vi "Autonomous Independent.vi"() -> ()   [LabVIEW 2018]
doc: "This VI is called when autonomous begins, and will automatically be terminated when autonomous ends. You can carry out timed or sensor driven robot movement independently without needing to return to the caller."
uses:
  <vilib>/Rock Robotics/WPI/DriverStation/WPI_DriverStationDerivedRobotMode.ctl
panel:
  out "ENCODER VALUE cLIMBER":dbl=20.0 format="%#_13g"
  out "ENCODER VALUE Retractor":dbl=20.0 format="%#_13g"
  out "ENCODER VALUE LIFT 2":dbl=20.0 format="%#_13g"
  out "ENCODER VALUE LIFT":dbl=20.0 format="%#_13g"
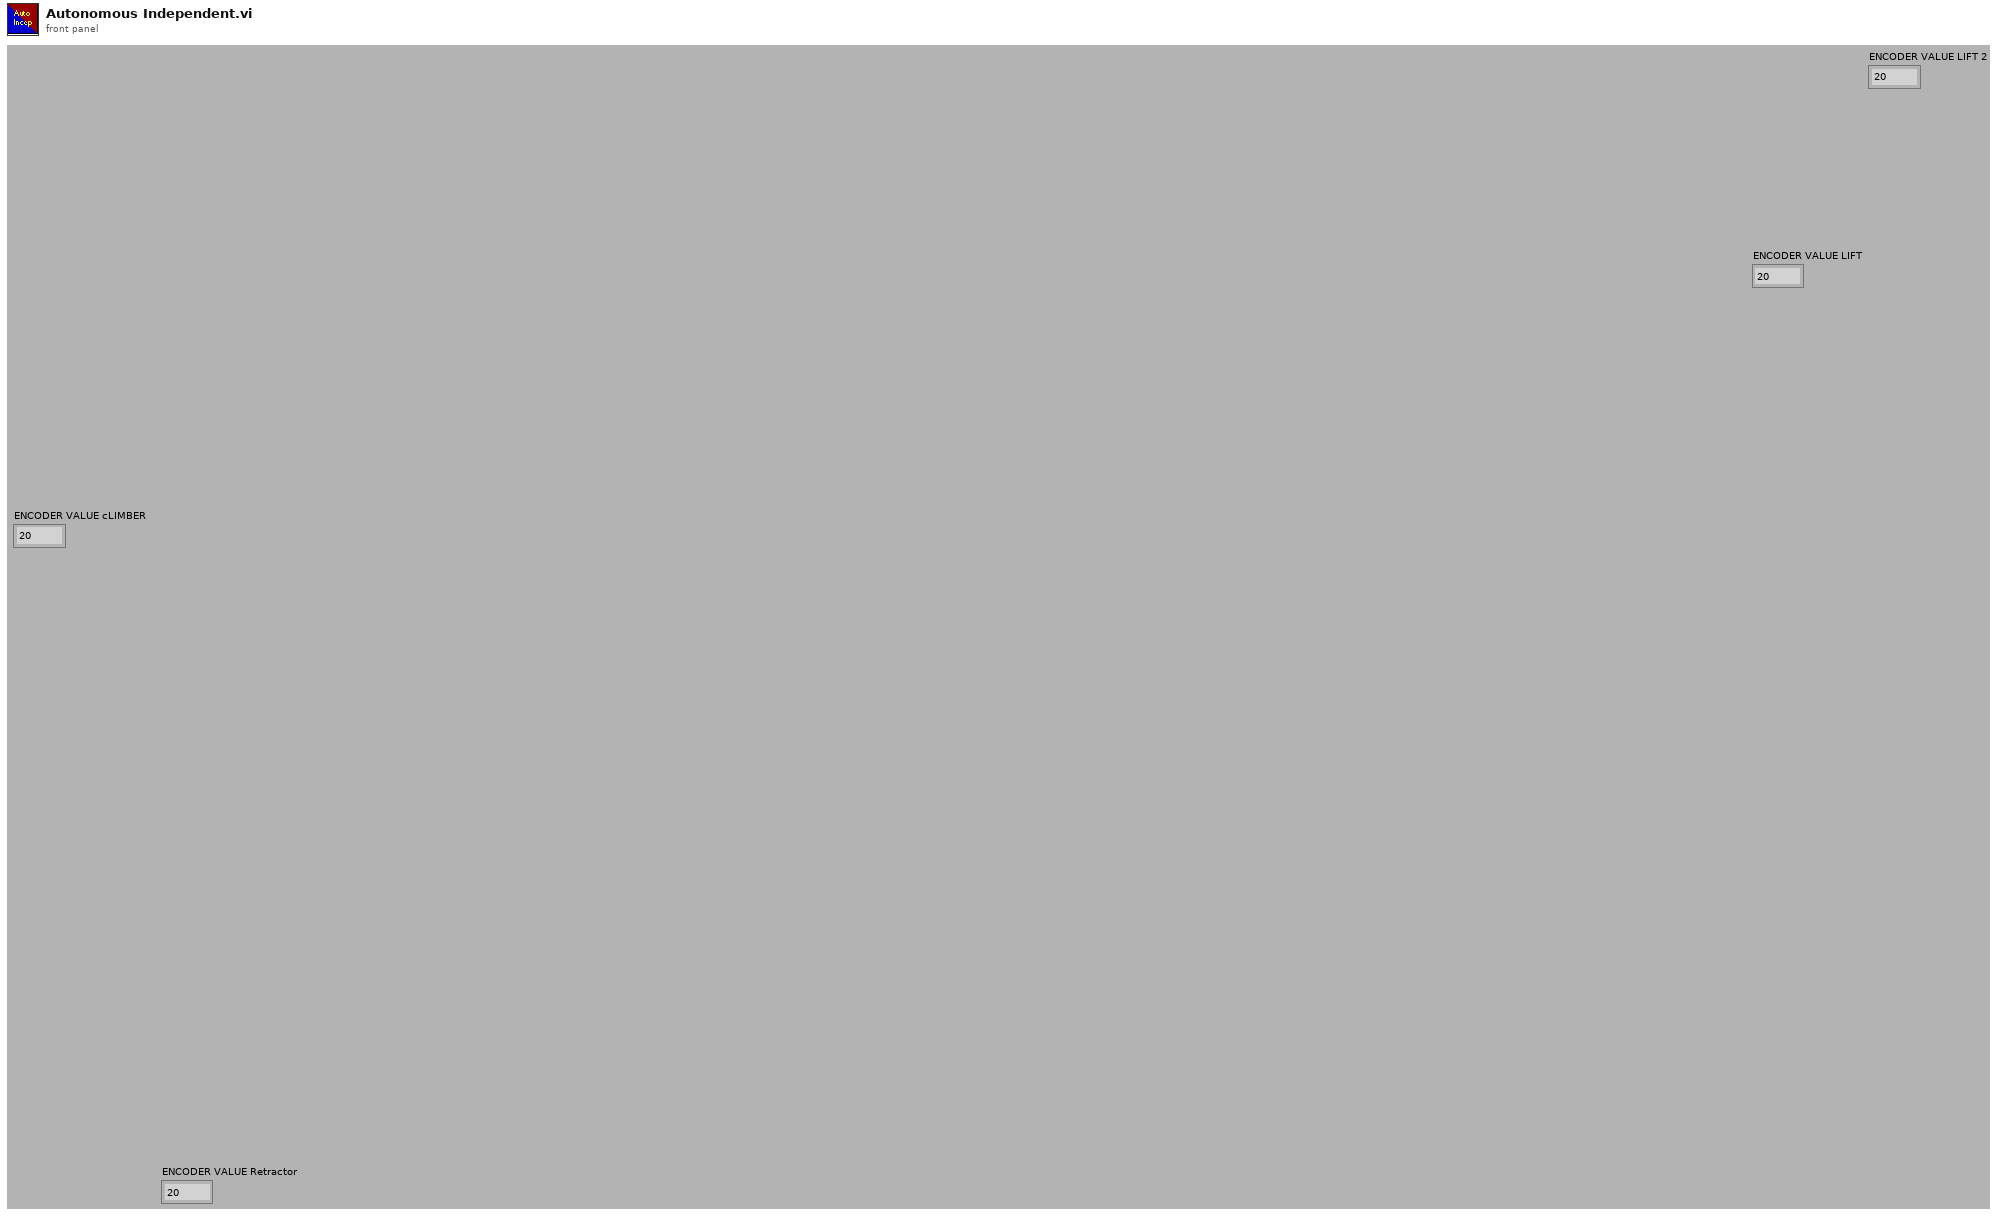
[diagram p1: front panel]
types:
  T1 = typedef "WPI_DriverStationDerivedRobotMode.ctl" = enum16{"Init", "Execute", "Stop"}
  T2 = typedef "WPI_JoystickDevRef.ctl" = cluster{"Device":T3}
  T3 = typedef "WPI_JoystickDeviceEnum.ctl" = enum16{"USB 0", "USB 1", "USB 2", "USB 3", "USB 4", "USB 5"}
  T4 = cluster{"Buttons[0]":bool, "Buttons[1]":bool, "Buttons[2]":bool, "Buttons[3]":bool, "Buttons[4]":bool, "Buttons[5]":bool, "Buttons[6]":bool, "Buttons[7]":bool, "Buttons[8]":bool, "Buttons[9]":bool}
  T5 = cluster{"Buttons[0]":bool, "Buttons[1]":bool, "Buttons[2]":bool, "Buttons[3]":bool, "Buttons[4]":bool, "Buttons[5]":bool, "Buttons[6]":bool, "Buttons[7]":bool, "Buttons[8]":bool, "Buttons[9]":bool, "Buttons[10]":bool, "Buttons[11]":bool}
  T6 = typedef "WPI_EncoderDevRef.ctl" = cluster{"DevStatus":errorcluster, "EncoderIndex":T7, "CounterIndex":T8, "DistancePerCount":dbl, "Decoding Type":T9}
  T7 = typedef "FPGA_EncoderIdx.ctl" = enum8{"Enc 0", "Enc 1", "Enc 2", "Enc 3", "Enc 4", "Enc 5", "Enc 6", "Enc 7", "Invalid"}
  T8 = typedef "FPGA_CounterCtrSystemIndex.ctl" = enum8{"Ctr 0", "Ctr 1", "Ctr 2", "Ctr 3", "Ctr 4", "Ctr 5", "Ctr 6", "Ctr 7", "Invalid"}
  T9 = typedef "WPI_EncoderType.ctl" = enum16{"1x", "2x", "4x"}
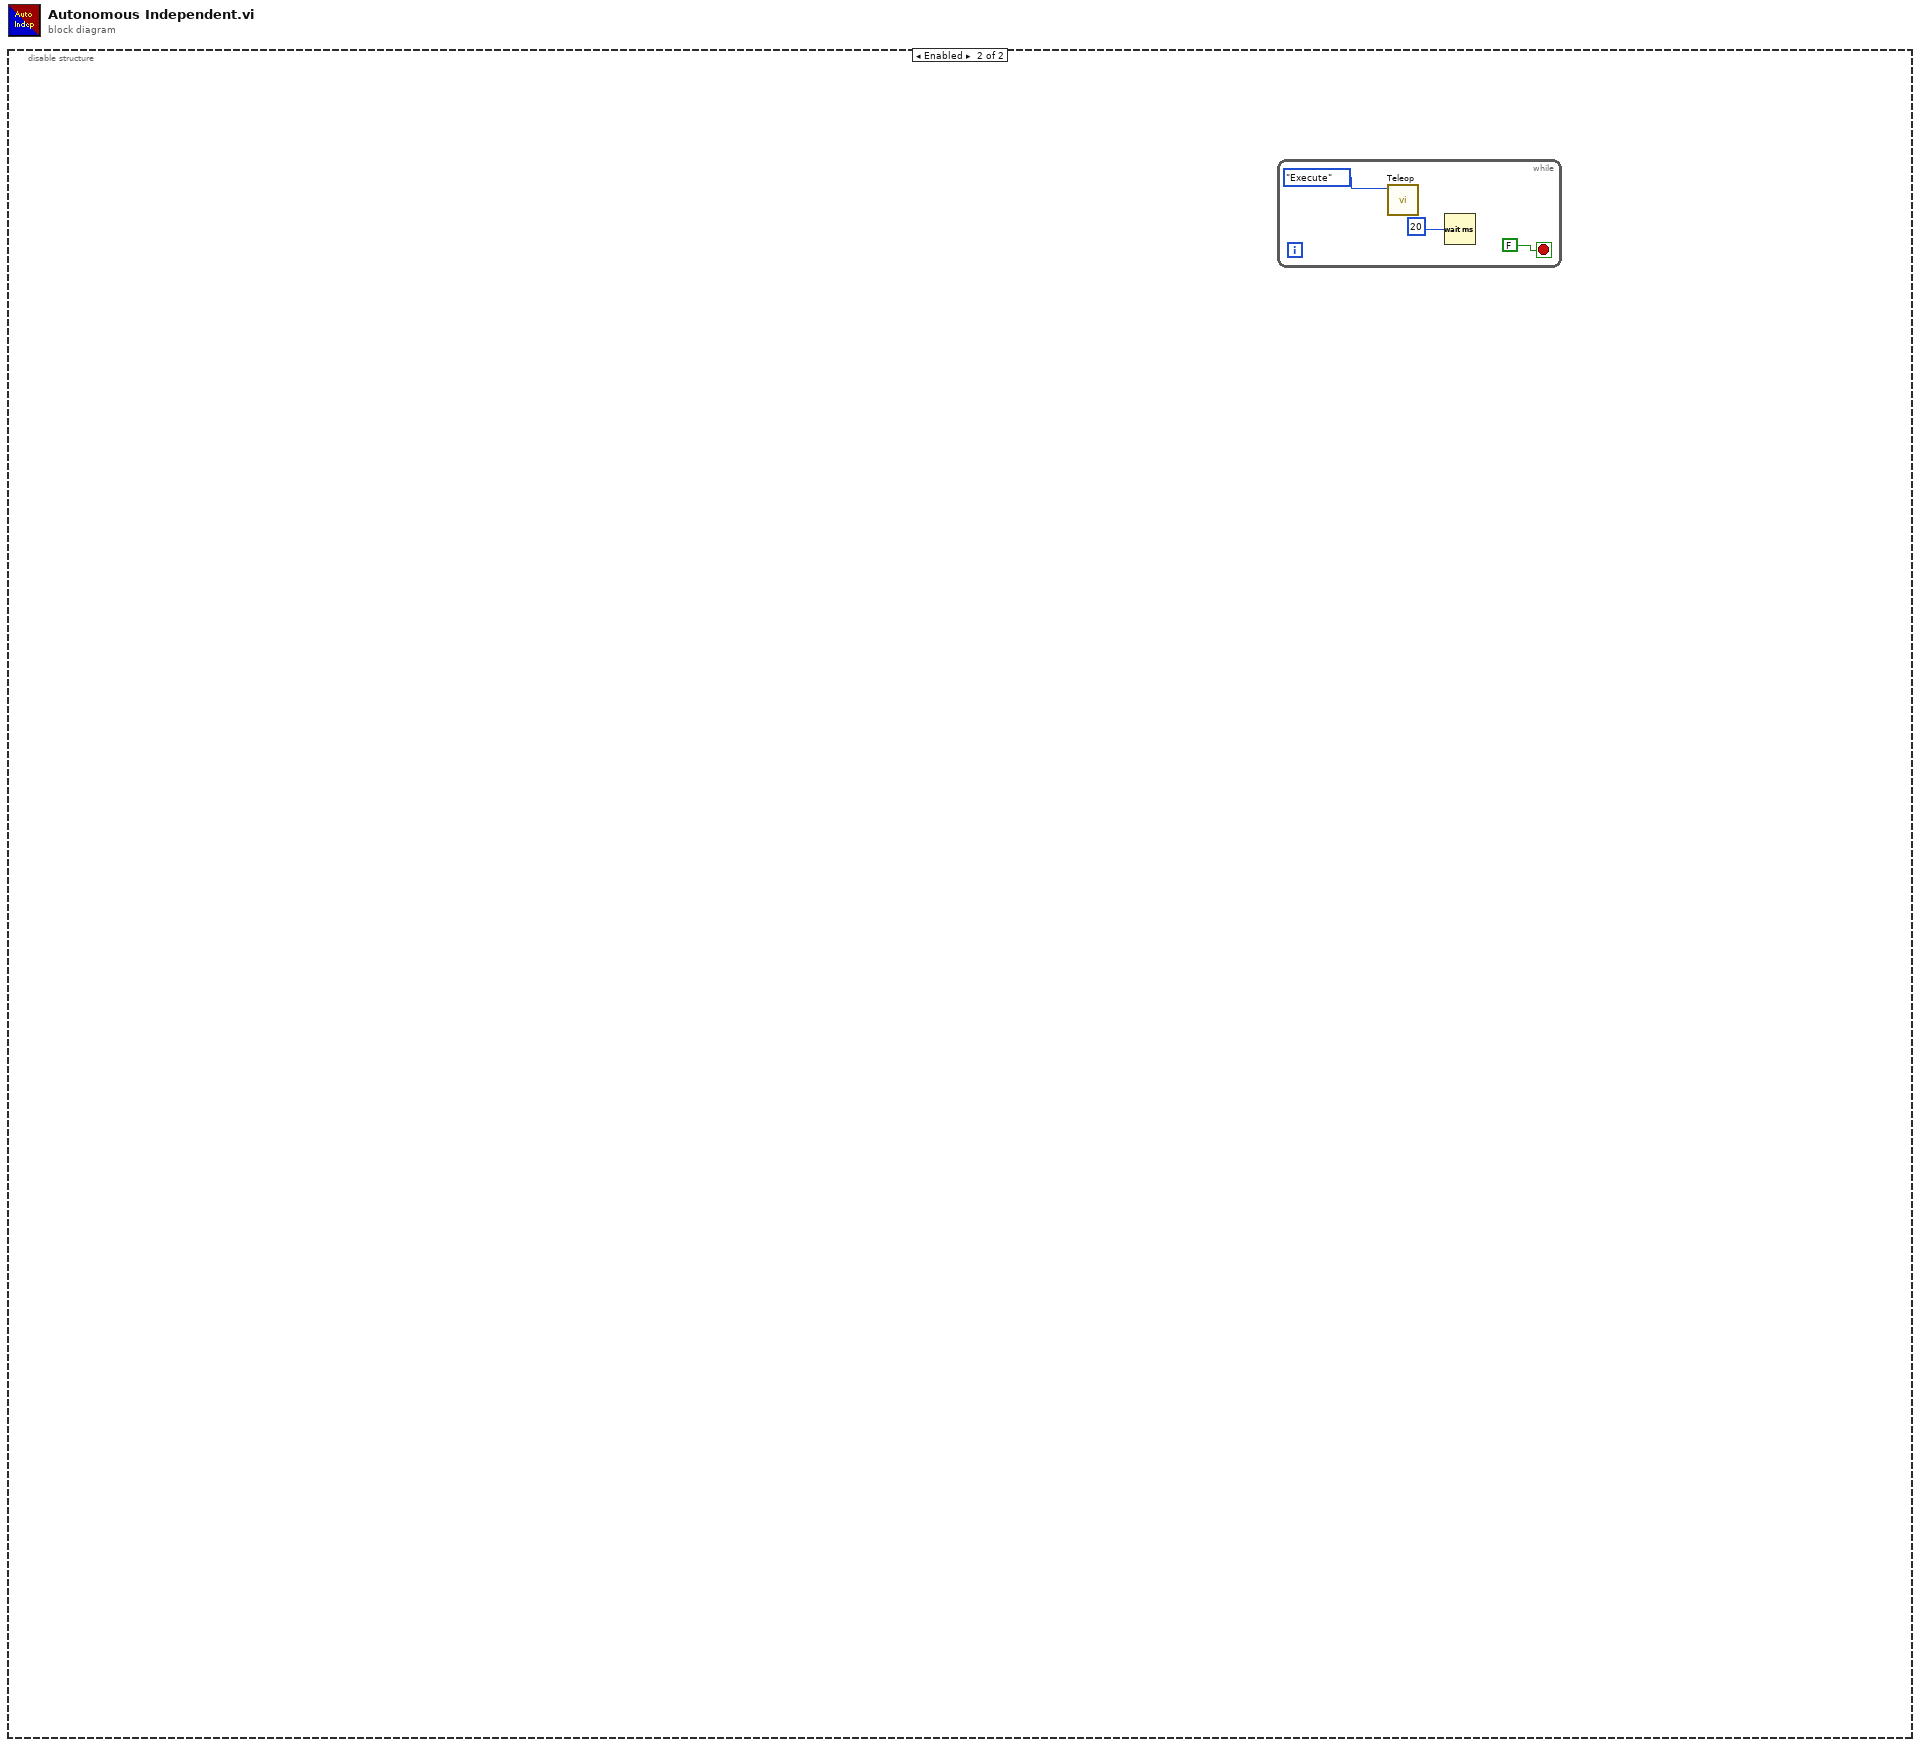
[diagram p0: block diagram]
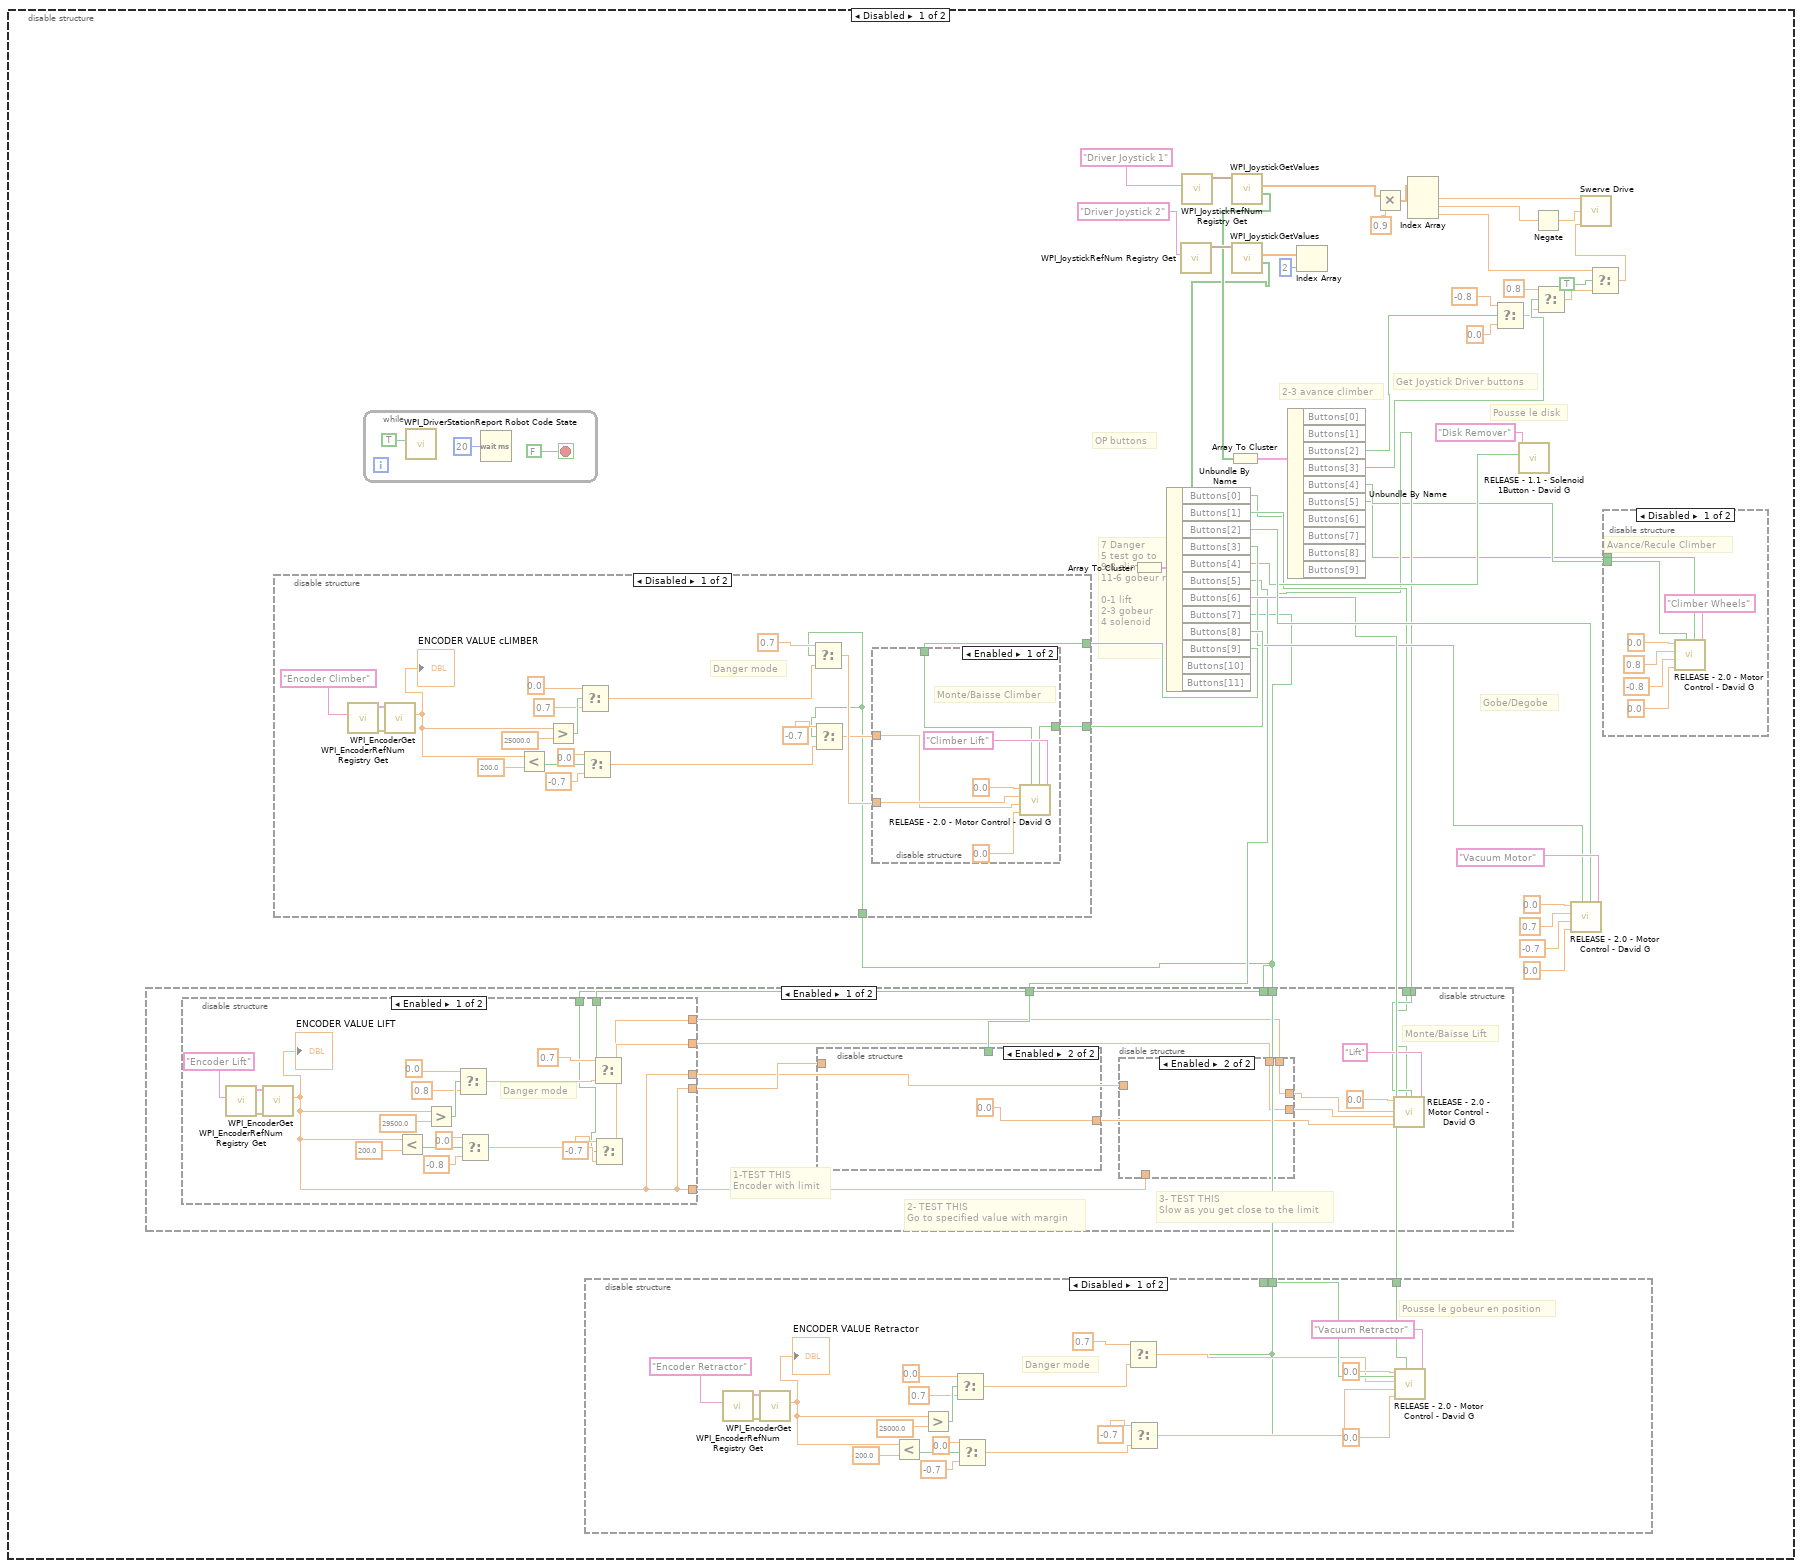
[diagram p2: hidden frame]
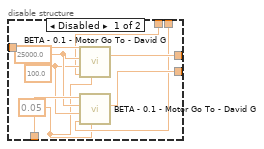
[diagram p7: hidden frame]
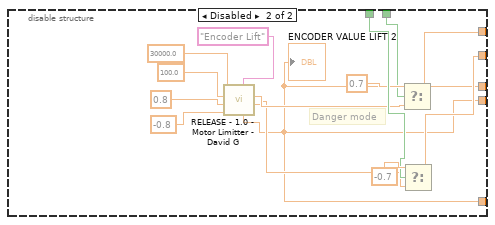
[diagram p8: hidden frame]
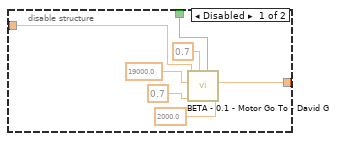
[diagram p9: hidden frame]
diagram:
  n1 = disable-structure shown="Enabled" {
    frame Disabled {
      # "2-3 avance climber"
      # "7 Danger\n5 test go to\n9-8 climber\n11-6 gobeur retractor\n\n0-1 lift\n2-3 gobeur\n4 solenoid"
      # "OP buttons"
      # "Gobe/Degobe"
      # "Pousse le disk"
      # "Get Joystick Driver buttons"
      n2 = while {
        stop <- FALSE stop-if-true
        n3 = call <vilib>:"WPI_DriverStationReport Robot Code State.vi"("Autonomous"=TRUE) -> ()  [unwired: 10 in, 1 out]
        n4 = Wait (ms)(milliseconds to wait=u32 20) -> ()  [unwired: 1 out]
      }
      n5 = call <vilib>:"WPI_JoystickRefNum Registry Get.vi"("refnum name"="Driver Joystick 2") -> ("JoystickDevRef"=w42:T2)  [unwired: 1 in, 9 out]
      n6 = call <vilib>:"WPI_JoystickRefNum Registry Get.vi"("refnum name"="Driver Joystick 1") -> ("JoystickDevRef"=w43:T2)  [unwired: 1 in, 9 out]
      n7 = call <vilib>:"WPI_JoystickGetValues.vi"("JoystickDevRef"=w43) -> ("Buttons"=w37:bool[], "Axes"=w38:dbl[])  [unwired: 6 in, 3 out]
      n8 = Array To Cluster(array=w37) -> (cluster=w36:T4)
      n9 = call <vilib>:"WPI_JoystickGetValues.vi"("JoystickDevRef"=w42) -> ("Buttons"=w28:bool[], "Axes"=w40:dbl[])  [unwired: 6 in, 3 out]
      n10 = Array To Cluster(array=w28) -> (cluster=w29:T5)
      n11 = Unbundle By Name(w29) -> ("Buttons[0]"=w14:bool, "Buttons[1]"=w15:bool, "Buttons[2]"=w27:bool, "Buttons[3]"=w19:bool, "Buttons[4]"=w16:bool, "Buttons[5]"=w18:bool, "Buttons[6]"=w20:bool, "Buttons[7]"=w17:bool, "Buttons[8]"=w21:bool, "Buttons[9]"=w22:bool)  [unwired: 2 out]
      n12 = disable-structure shown="Enabled" {
        disable-tunnel: w14 -> [w117 _]
        disable-tunnel: w15 -> [w116 _]
        disable-tunnel: w17 -> [w114 _]
        disable-tunnel: w17 -> [w113 _]
        disable-tunnel: w18 -> [w111 _]
        frame Enabled {
          # "3- TEST THIS\nSlow as you get close to the limit"
          # "1-TEST THIS\nEncoder with limit"
          # "2- TEST THIS \nGo to specified value with margin"
          # "Monte/Baisse Lift"
          n13 = disable-structure shown="Enabled" {
            disable-tunnel: [w136 w159] -> w107
            disable-tunnel: [w135 w160] -> w108
            disable-tunnel: w114 -> [w134 w152]
            disable-tunnel: w113 -> [w131 w162]
            disable-tunnel: [w130 w150] -> w112
            disable-tunnel: [w130 w150] -> w105
            disable-tunnel: [w130 w150] -> w104
            frame Enabled {
              # "Danger mode"
              n14 = call <vilib>:"WPI_EncoderRefNum Registry Get.vi"("refnum name"="Encoder Lift") -> ("error out"=w149:errorcluster, "EncoderDevRef"=w148:T6)  [unwired: 9 in]
              n15 = call <vilib>:"WPI_EncoderGet.vi"("error in (no error)"=w149, "EncoderDevRef"=w148) -> ("Distance"=w130:dbl)  [unwired: 4 in, 5 out]
              "ENCODER VALUE LIFT" <- w130
              n16 = Less?(x=w130, y=200.0 ("f")) -> (x < y?=w143:bool)
              n17 = Greater?(x=w130, y=29500.0 ("f")) -> (0:w144:bool)
              n18 = Select(t=0.0 ("f"), s=w144, f=0.8) -> (s? t:f=w138:dbl)
              n19 = Select(t=0.0 ("f"), s=w143, f=-0.8) -> (s? t:f=w137:dbl)
              n20 = Select(t=0.7 ("f"), s=w134, f=w138) -> (s? t:f=w135:dbl)
              n21 = Select(t=-0.7 ("f"), s=w131, f=w137) -> (s? t:f=w136:dbl)
            }
            frame Disabled {
              # "Danger mode"
              n22 = call "RELEASE - 1.0 - Motor Limitter - David G.vi"("refnum name"="Encoder Lift", "Backward Speed"=-0.8 ("f"), "Forward Speed"=0.8 ("f"), "Backward Limit"=100.0 ("f"), "Forward Limit"=30000.0 ("f")) -> ("Backward Value"=w157:dbl, "Forward Value"=w158:dbl, "Encoder Value"=w150:dbl)  [unwired: 4 in]
              "ENCODER VALUE LIFT 2" <- w150
              n23 = Select(t=0.7 ("f"), s=w152, f=w158) -> (s? t:f=w160:dbl)
              n24 = Select(t=-0.7 ("f"), s=w162, f=w157) -> (s? t:f=w159:dbl)
            }
          }
          n25 = disable-structure shown="Enabled" {
            disable-tunnel: w112 -> [w167 _]
            disable-tunnel: w111 -> [w166 _]
            disable-tunnel: [w165 0.0 ("f")] -> w110
            frame Disabled {
              n26 = call "BETA - 0.1 - Motor Go To - David G.vi"("Encoder Value"=w167, "Go To"=19000.0 ("f"), "Speed"=0.7 ("f"), "Default Neutral Speed"=0.7 ("f"), "Button"=w166, "Margin (Nullable)"=2000.0 ("f")) -> ("Output Neutral Speed"=w165:dbl)  [unwired: 4 in]
            }
            frame Enabled {
            }
          }
          n27 = disable-structure shown="Enabled" {
            disable-tunnel: [w126 w129] -> w109
            disable-tunnel: w108 -> [w125 w129]
            disable-tunnel: w107 -> [w120 w128]
            disable-tunnel: [w127 w128] -> w106
            disable-tunnel: w105 -> [w124 _]
            disable-tunnel: w104 -> [w123 _]
            frame Disabled {
              w119 = 0.05 ("f")
              w121 = 100.0 ("f")
              w122 = 25000.0 ("f")
              n28 = call "BETA - 0.1 - Motor Go To - David G.vi"("Encoder Value"=w124, "Go To"=w122, "Speed"=w120, "Default Neutral Speed"=w119, "Margin (Nullable)"=w121) -> ("Output Neutral Speed"=w126:dbl)  [unwired: 5 in]
              n29 = call "BETA - 0.1 - Motor Go To - David G.vi"("Encoder Value"=w123, "Go To"=w122, "Speed"=w125, "Default Neutral Speed"=w119, "Margin (Nullable)"=w121) -> ("Output Neutral Speed"=w127:dbl)  [unwired: 5 in]
            }
            frame Enabled {
            }
          }
          n30 = call "RELEASE - 2.0 - Motor Control - David G.vi"("refnum name"="Lift", "Bouton Arrière"=w117, "Bouton Avant"=w116, "FF"=w110, "FT"=w106, "TF"=w109, "TT"=0.0 ("f")) -> ()  [unwired: 5 in]
        }
        frame Disabled {
        }
      }
      n31 = disable-structure shown="Disabled" {
        disable-tunnel: w17 -> [w54 _]
        disable-tunnel: w21 -> [w53 _]
        disable-tunnel: w22 -> [w52 _]
        frame Disabled {
          # "Danger mode"
          n32 = call <vilib>:"WPI_EncoderRefNum Registry Get.vi"("refnum name"="Encoder Climber") -> ("error out"=w72:errorcluster, "EncoderDevRef"=w71:T6)  [unwired: 9 in]
          n33 = call <vilib>:"WPI_EncoderGet.vi"("error in (no error)"=w72, "EncoderDevRef"=w71) -> ("Distance"=w61:dbl)  [unwired: 4 in, 5 out]
          "ENCODER VALUE cLIMBER" <- w61
          n34 = Less?(x=w61, y=200.0 ("f")) -> (x < y?=w66:bool)
          n35 = Greater?(x=w61, y=25000.0 ("f")) -> (0:w67:bool)
          n36 = Select(t=0.0 ("f"), s=w67, f=0.7) -> (s? t:f=w60:dbl)
          n37 = Select(t=0.0 ("f"), s=w66, f=-0.7) -> (s? t:f=w59:dbl)
          n38 = Select(t=0.7 ("f"), s=w54, f=w60) -> (s? t:f=w56:dbl)
          n39 = Select(t=-0.7 ("f"), s=w54, f=w59) -> (s? t:f=w55:dbl)
          n40 = disable-structure shown="Enabled" {
            disable-tunnel: w52 -> [w76 _]
            disable-tunnel: w53 -> [w75 _]
            disable-tunnel: w56 -> [w74 _]
            disable-tunnel: w55 -> [w73 _]
            frame Enabled {
              # "Monte/Baisse Climber"
              n41 = call "RELEASE - 2.0 - Motor Control - David G.vi"("refnum name"="Climber Lift", "Bouton Arrière"=w75, "Bouton Avant"=w76, "FF"=0.0 ("f"), "FT"=w73, "TF"=w74, "TT"=0.0 ("f")) -> ()  [unwired: 5 in]
            }
            frame Disabled {
            }
          }
        }
        frame Enabled {
        }
      }
      n42 = disable-structure shown="Disabled" {
        disable-tunnel: _ -> [w100 _]
        disable-tunnel: w17 -> [w81 _]
        disable-tunnel: w20 -> [w80 _]
        frame Disabled {
          # "Danger mode"
          # "Pousse le gobeur en position"
          n43 = call <vilib>:"WPI_EncoderRefNum Registry Get.vi"("refnum name"="Encoder Retractor") -> ("error out"=w99:errorcluster, "EncoderDevRef"=w98:T6)  [unwired: 9 in]
          n44 = call <vilib>:"WPI_EncoderGet.vi"("error in (no error)"=w99, "EncoderDevRef"=w98) -> ("Distance"=w88:dbl)  [unwired: 4 in, 5 out]
          "ENCODER VALUE Retractor" <- w88
          n45 = Less?(x=w88, y=200.0 ("f")) -> (x < y?=w93:bool)
          n46 = Greater?(x=w88, y=25000.0 ("f")) -> (0:w94:bool)
          n47 = Select(t=0.0 ("f"), s=w94, f=0.7) -> (s? t:f=w87:dbl)
          n48 = Select(t=0.0 ("f"), s=w93, f=-0.7) -> (s? t:f=w86:dbl)
          n49 = Select(t=0.7 ("f"), s=w81, f=w87) -> (s? t:f=w83:dbl)
          n50 = Select(t=-0.7 ("f"), s=w81, f=w86) -> (s? t:f=w82:dbl)
          n51 = call "RELEASE - 2.0 - Motor Control - David G.vi"("refnum name"="Vacuum Retractor", "Bouton Arrière"=w100, "Bouton Avant"=w80, "FF"=0.0 ("f"), "FT"=w82, "TF"=w83, "TT"=0.0 ("f")) -> ()  [unwired: 5 in]
        }
        frame Enabled {
        }
      }
      n52 = Unbundle By Name(w36) -> ("Buttons[2]"=w11:bool, "Buttons[3]"=w10:bool, "Buttons[4]"=w13:bool, "Buttons[5]"=w12:bool)  [unwired: 6 out]
      n53 = Index Array(array=w40, index=2) -> ()  [unwired: 1 out]
      n54 = Multiply(x=w38, y=0.9) -> (x*y=w23:dbl[])
      n55 = Index Array(array=w23) -> (element #1=w1:dbl, element #2=w25:dbl, element #3=w4:dbl)  [unwired: 3 in]
      n56 = Select(t=-0.8 ("y"), s=w11, f=0.0 ("y")) -> (s? t:f=w9:dbl)
      n57 = call "RELEASE - 1.1 - Solenoid 1Button - David G.vi"(10:w16, "refnum name"="Disk Remover") -> ()  [unwired: 10 in]
      n58 = Negate(x=w25) -> (-x=w26:dbl)
      n59 = Select(t=0.8 ("y"), s=w10, f=w9) -> (s? t:f=w5:dbl)
      n60 = call "RELEASE - 2.0 - Motor Control - David G.vi"("refnum name"="Vacuum Motor", "Bouton Arrière"=w27, "Bouton Avant"=w19, "FF"=0.0 ("f"), "FT"=-0.7 ("f"), "TF"=0.7 ("f"), "TT"=0.0 ("f")) -> ()  [unwired: 5 in]
      n61 = Select(t=w4, s=TRUE, f=w5) -> (s? t:f=w3:dbl)
      n62 = call "Swerve Drive.vi"("X"=w1, "Y"=w26, "Z"=w3) -> ()  [unwired: 13 in]
      n63 = disable-structure shown="Disabled" {
        disable-tunnel: w12 -> [w46 _]
        disable-tunnel: w13 -> [w45 _]
        frame Disabled {
          # "Avance/Recule Climber"
          n64 = call "RELEASE - 2.0 - Motor Control - David G.vi"("refnum name"="Climber Wheels", "Bouton Arrière"=w46, "Bouton Avant"=w45, "FF"=0.0 ("f"), "FT"=-0.8 ("f"), "TF"=0.8 ("f"), "TT"=0.0 ("f")) -> ()  [unwired: 5 in]
        }
        frame Enabled {
        }
      }
    }
    frame Enabled {
      n65 = while {
        stop <- FALSE stop-if-true
        n66 = call "Teleop.vi"("Call Context"=WPI_DriverStationDerivedRobotMode."Execute") -> ()  [unwired: 11 in]
        n67 = Wait (ms)(milliseconds to wait=20) -> ()  [unwired: 1 out]
      }
    }
  }
